vi "FT10_Read LVM Files & Auto Save.vi"() -> ()   [LabVIEW 2015]
uses:
  <vilib>/Waveform/WDTOps.llb/WDT Waveform Duration DBL.vi
panel:
  out "Y min":dbl format="%0.2f"
  out "Y max":dbl format="%0.2f"
  out "X Max":dbl format="%0.2f"
  in  "Y Scale.Range:Maximum":dbl
  in  "Y Scale.Range:Minimum":dbl
  in  "X Scale.Range:Maximum":dbl
  in  "X Scale.Range:Minimum":dbl
  out "Waveform Graph":dynamicdata(graph)
  in  "LVM File":path[](array[path]) caption="Filename"
  in  "PNG save file":path[](array[path])
  in  "JPEG save file":path[](array[path])
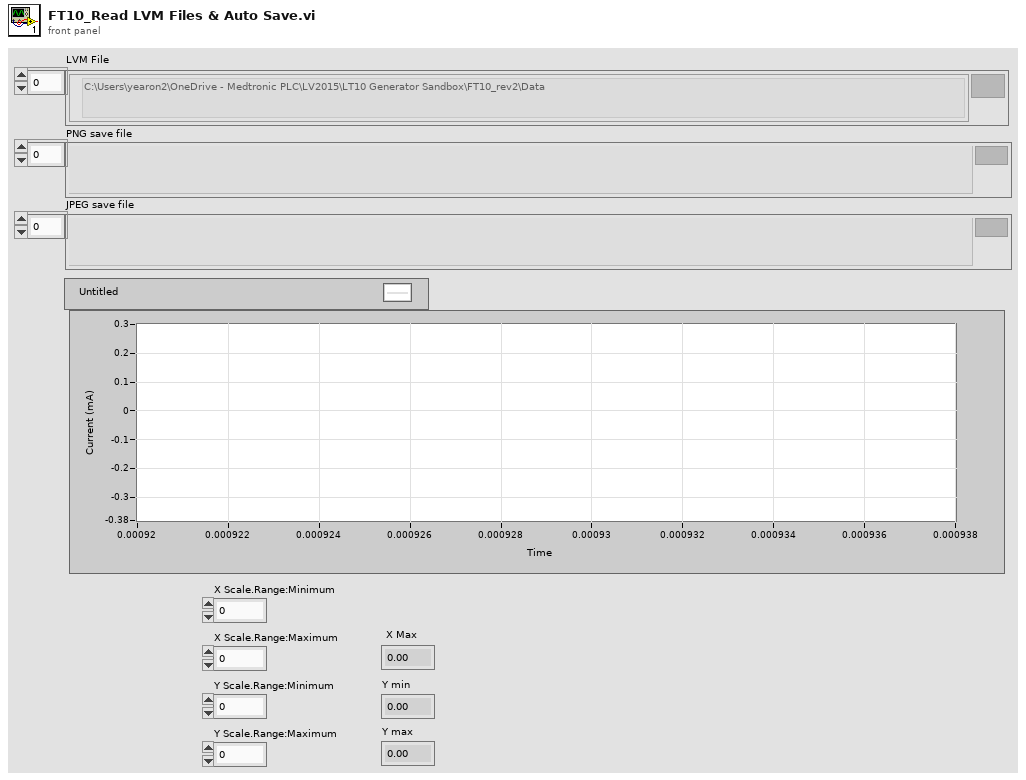
[diagram p1: front panel]
types:
  T1 = typedef "imagedata.ctl" = cluster{"image type":i32, "image depth":i32, "image":u8[], "mask":u8[], "colors":u32[], "Rectangle":cluster{"left":i16, "top":i16, "right":i16, "bottom":i16}}
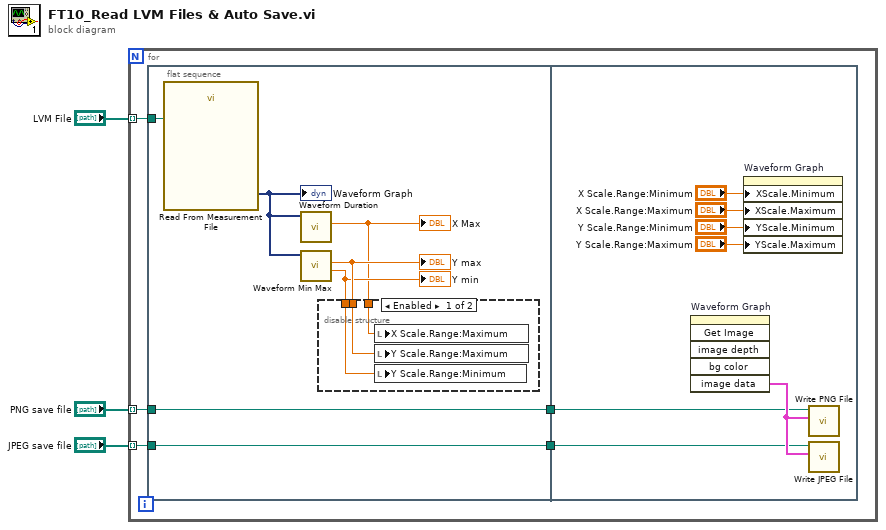
[diagram p0: block diagram]
diagram:
  n1 = for {
    tunnel: "LVM File" -> [w8] mode=indexing
    tunnel: "PNG save file" -> [w6] mode=indexing
    tunnel: "JPEG save file" -> [w4] mode=indexing
    n2 = flat-sequence {
      tunnel: w8 -> [w11]
      tunnel: [w10] -> w7
      tunnel: w6 -> [w10]
      tunnel: [w9] -> w5
      tunnel: w4 -> [w9]
      tunnel: w7 -> [w20]
      tunnel: w5 -> [w19]
      frame #0 {
        n3 = call "Read From Measurement File"("Filename"=w11) -> ("Signals"=w15:dynamicdata)  [unwired: 5 in, 5 out]
        "Waveform Graph" <- w15
        n4 = call-poly <vilib>:"Waveform Duration.vi"("waveform in"=w15) -> ("duration"=w12:dbl)  [unwired: 8 in, 2 out]
        "X Max" <- w12
        n5 = call <vilib>:"Waveform Min Max.vi"("waveform in"=w15) -> ("Y min"=w13:dbl, "Y max"=w14:dbl)  [unwired: 5 in, 4 out]
        "Y max" <- w14
        "Y min" <- w13
        n6 = disable-structure shown="Enabled" {
          disable-tunnel: w14 -> [w18 _]
          disable-tunnel: w13 -> [w17 _]
          disable-tunnel: w12 -> [w16 _]
          frame Enabled {
            n7 = local write "X Scale.Range:Maximum"(w16) -> ()
            n8 = local write "Y Scale.Range:Maximum"(w18) -> ()
            n9 = local write "Y Scale.Range:Minimum"(w17) -> ()
          }
          frame Disabled {
          }
        }
      }
      frame #1 {
        n10 = invoke on="Waveform Graph" class="WFGraph (strict)" method="Get Image"() -> ("image data"=w25:T1)  [unwired: 6 in, 5 out]
        n11 = property on="Waveform Graph" class="WFGraph (strict)"("XScale.Minimum"="X Scale.Range:Minimum", "XScale.Maximum"="X Scale.Range:Maximum", "YScale.Minimum"="Y Scale.Range:Minimum", "YScale.Maximum"="Y Scale.Range:Maximum") -> ()  [unwired: 2 in, 2 out]
        n12 = call <vilib>:"Write PNG File.vi"("image data"=w25, "path to PNG file"=w20) -> ()  [unwired: 8 in, 2 out]
        n13 = call <vilib>:"Write JPEG File.vi"("image data"=w25, "path to JPEG file"=w19) -> ()  [unwired: 8 in, 2 out]
      }
    }
  }
